vi "F_ILS_FTS.vi"(0 "ilsextent":dbl=50.0, 1 "vStart":dbl=5987.0, 2 "OPD":dbl=1.8, 3 "FOV":dbl=0.00296, 4 "vEnd":dbl=6165.0, 5 "modulation_loss":dbl=0.025) -> (7 "Total":T1(graph))   [LabVIEW 2010]
uses:
  <vilib>/Analysis/1siggen.llb/Ramp Pattern by Delta.vi
  <vilib>/Analysis/NI_AALBase.lvlib
panel:
  out "Align":T1(graph)
  out "Aperture":T1(graph)
  out "OPD":T1(graph)
  in  "common_grid resolution":dbl=0.01
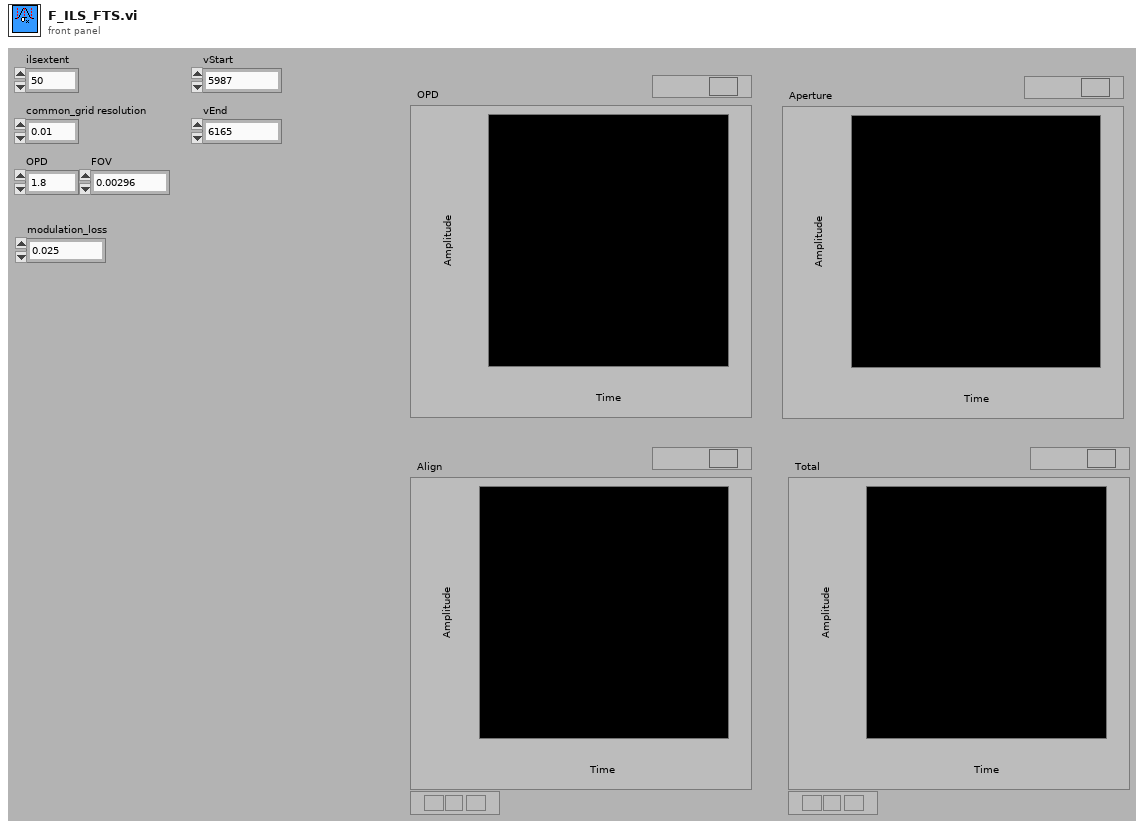
[diagram p1: front panel]
types:
  T1 = cluster{"Ramp Pattern":dbl[], "Sinc Pattern":dbl[]}
  T2 = cluster{"Ramp Pattern":dbl[], "Pulse Pattern":dbl[]}
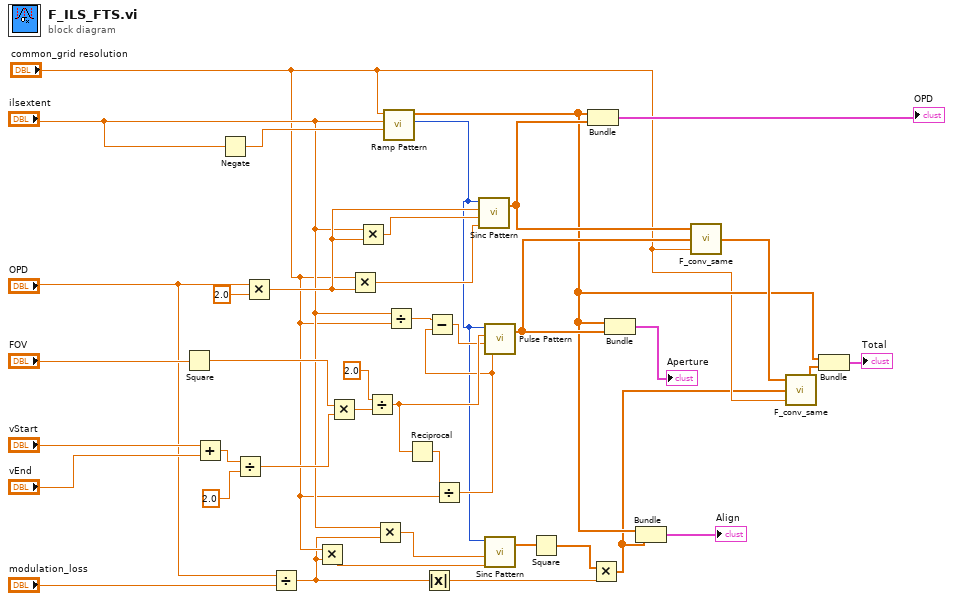
[diagram p0: block diagram]
diagram:
  n1 = Square(x="FOV") -> (x^2=w30:dbl)
  n2 = Add(x="vStart", y="vEnd") -> (x+y=w32:dbl)
  n3 = Negate(x="ilsextent") -> (-x=w40:dbl)
  n4 = Divide(x=w32, y=2.0) -> (x/y=w29:dbl)
  n5 = Multiply(x="OPD", y=2.0) -> (x*y=w36:dbl)
  n6 = Divide(x="OPD", y="modulation_loss") -> (x/y=w4:dbl)
  n7 = Multiply(x="common_grid resolution", y=w4) -> (x*y=w18:dbl)
  n8 = Multiply(x=w30, y=w29) -> (x*y=w28:dbl)
  n9 = Multiply(x="common_grid resolution", y=w36) -> (x*y=w38:dbl)
  n10 = Multiply(x="ilsextent", y=w36) -> (x*y=w37:dbl)
  n11 = Divide(x=2.0 ("y"), y=w28) -> (x/y=w26:dbl)
  n12 = Multiply(x="ilsextent", y=w4) -> (x*y=w16:dbl)
  n13 = call-poly <vilib>:"Ramp Pattern.vi"("start"=w40, "end"="ilsextent", "delta"="common_grid resolution") -> ("samples"=w21:i32, "Ramp Pattern"=w6:dbl[])  [unwired: 6 in, 1 out]
  n14 = Divide(x="ilsextent", y="common_grid resolution") -> (x/y=w24:dbl)
  n15 = Reciprocal(x=w26) -> (1/x=w25:dbl)
  n16 = Absolute Value(x=w4) -> (abs(x)=w3:dbl)
  n17 = Divide(x=w25, y="common_grid resolution") -> (x/y=w23:dbl)
  n18 = Subtract(x=w24, y=w23) -> (x-y=w22:dbl)
  n19 = call <vilib>:"Sinc Pattern.vi"("delta t"=w38, "delay"=w37, "amplitude"=w36, "samples"=w21) -> ("Sinc Pattern"=w14:dbl[])  [unwired: 1 out]
  n20 = call <vilib>:"Pulse Pattern.vi"("width"=w23, "delay"=w22, "amplitude"=w26, "samples"=w21) -> ("Pulse Pattern"=w11:dbl[])  [unwired: 1 out]
  n21 = call <vilib>:"Sinc Pattern.vi"("delta t"=w18, "delay"=w16, "samples"=w21) -> ("Sinc Pattern"=w15:dbl[])  [unwired: 1 in, 1 out]
  n22 = Square(x=w15) -> (x^2=w2:dbl[])
  n23 = Bundle("Ramp Pattern"=w6, "Sinc Pattern"=w14) -> (→"OPD":T1)  [unwired: 1 in]
  n24 = Multiply(x=w2, y=w3) -> (x*y=w1:dbl[])
  n25 = Bundle("Ramp Pattern"=w6, "Pulse Pattern"=w11) -> (→"Aperture":T2)  [unwired: 1 in]
  n26 = Bundle("Ramp Pattern"=w6, w1) -> (→"Align":cluster{"Ramp Pattern":dbl[], dbl[]})  [unwired: 1 in]
  n27 = call "F_conv_same.vi"("dt"="common_grid resolution", "Pulse Pattern"=w11, "Sinc Pattern"=w14) -> ("Convolved"=w9:dbl[])
  n28 = call "F_conv_same.vi"("dt"="common_grid resolution", "Pulse Pattern"=w1, "Sinc Pattern"=w9) -> ("Convolved"=w7:dbl[])
  n29 = Bundle("Ramp Pattern"=w6, "Convolved"=w7) -> (→"Total":cluster{"Ramp Pattern":dbl[], "Convolved":dbl[]})  [unwired: 1 in]
